vi "regCmd.vi"(8 "error in (no error)":errorcluster, 10 "cmdReg":string[](array[string]), 11 "tcpServer in":refnum<class "TcpServer.lvclass">) -> (0 "error out":errorcluster, 3 "tcpServer out":refnum<class "TcpServer.lvclass">)   [LabVIEW 2018, in "TcpServer.lvclass"]
doc: "Inform the TCP Server which commands are registered and allowed to be used by LabVIEW Component."
uses:
  TcpServer.lvclass
  TcpServer.lvclass/TcpServer.ctl
  TcpServerCmd/TcpServerCmd.lvclass/TcpServerCmd.ctl
  TcpServerCmd/TcpServerCmd.lvclass
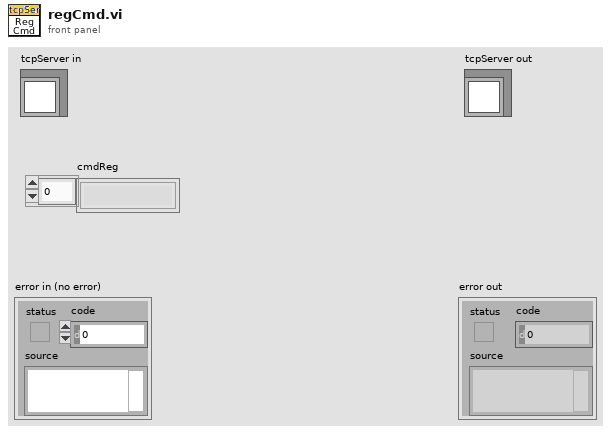
[diagram p1: front panel]
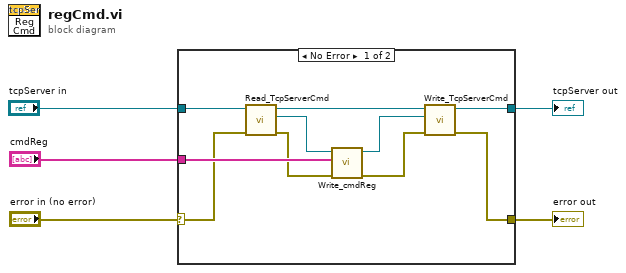
[diagram p0: block diagram]
diagram:
  n1 = case shown="No Error" "error in (no error)" {
    selector: "error in (no error)" -> [w11 w17]
    tunnel: [w6 w17] -> w4
    tunnel: [w9 w16] -> w2
    tunnel: "tcpServer in" -> [w14 w16]
    tunnel: "cmdReg" -> [w15 _]
    frame No Error {
      n2 = call "Read_TcpServerCmd.vi"("error in (no error)"=w11, "TcpServer in"=w14) -> ("error out"=w10:errorcluster, "TcpServerCmd.lvclass"=w13:refnum<class "TcpServerCmd.lvclass">, "TcpServer out"=w12:refnum<class "TcpServer.lvclass">)  [unwired: 7 in]
      n3 = call "Write_cmdReg.vi"("error in (no error)"=w10, "cmdReg"=w15, "TcpServerCmd in"=w13) -> ("error out"=w7:errorcluster, "TcpServerCmd out"=w8:refnum<class "TcpServerCmd.lvclass">)  [unwired: 7 in]
      n4 = call "Write_TcpServerCmd.vi"("error in (no error)"=w7, "TcpServerCmd.lvclass"=w8, "TcpServer in"=w12) -> ("error out"=w6:errorcluster, "TcpServer out"=w9:refnum<class "TcpServer.lvclass">)  [unwired: 7 in]
    }
    frame Error {
    }
  }
  "error out" <- w4
  "tcpServer out" <- w2
